vi "velx.vi"() -> (3 "function return":dbl)   [LabVIEW 2017, in "HapticSTM.lvlib"]
doc: "extern \"C\" __declspec(dllexport) double velx();"
uses:
  <userlib>/HapticSTM/Feedbackless - Testdata/HapticSTM_Feedblackless_testdata Folder/HapticSTM.lvlib
  <userlib>/HapticSTM/HapticSTM.dll
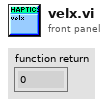
[diagram p1: front panel]
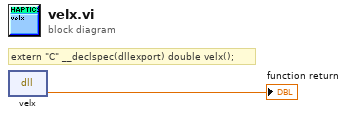
[diagram p0: block diagram]
diagram:
  # "extern \"C\" __declspec(dllexport) double velx();"
  n1 = dll-call lib="C:/Program Files/National Instruments/LabVIEW 2019/user.lib/HapticSTM/HapticSTM.*" fn="velx"() -> (→"function return":dbl)  [unwired: 3 in, 2 out]
